vi "cv_08_02.vi"() -> ()   [LabVIEW 2013]
uses:
  <vilib>/Utility/file.llb/Write To Spreadsheet File (DBL).vi
  <vilib>/Analysis/NI_AALBase.lvlib
panel:
  out "Table":string[][](table)
  out "Waveform Graph":dbl[][](graph)
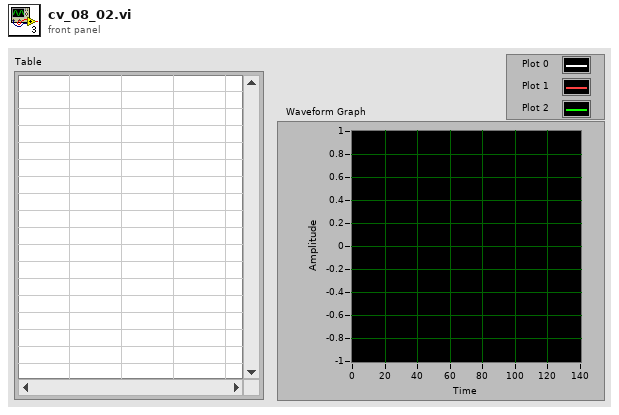
[diagram p1: front panel]
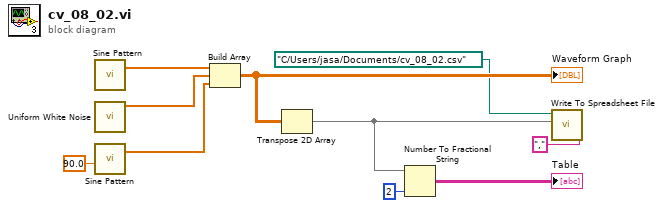
[diagram p0: block diagram]
diagram:
  n1 = call <vilib>:"Sine Pattern.vi"() -> ("Sinusoidal Pattern"=w9:dbl[])  [unwired: 4 in, 1 out]
  n2 = call <vilib>:"Uniform White Noise.vi"() -> ("uniform white noise"=w8:dbl[])  [unwired: 10 in, 1 out]
  n3 = call <vilib>:"Sine Pattern.vi"("phase(degrees)"=90.0) -> ("Sinusoidal Pattern"=w7:dbl[])  [unwired: 3 in, 1 out]
  n4 = Build Array(w9, w8, w7) -> (w6:dbl[][])
  "Waveform Graph" <- w6
  n5 = Transpose 2D Array(2D array=w6) -> (transposed array=w5:dbl[][])
  n6 = Number To Fractional String(number=w5, precision (6)=2) -> (F-format string=→"Table":string[][])  [unwired: 2 in]
  n7 = call-poly <vilib>:"Write To Spreadsheet File.vi"("delimiter (\\t)"=",", "2D data"=w5, "file path (dialog if empty)"=path "C:/Users/jasa/Documents/cv_08_02.csv") -> ()  [unwired: 5 in, 1 out]
